vi "Fit Controls to Rect.vi"(4 "Error In":errorcluster, 6 "Rect":T1, 7 "GObjs":refnum<vi>[](array[refnum])) -> (0 "Error Out":errorcluster, 3 "GObjs":refnum<vi>[](array[refnum]))   [LabVIEW 2017]
doc: "Moves the front panel objects in GObjs so that their combined bounding rectangle is centred inside Rect."
uses:
  <vilib>/Utility/miscctls.llb/LVRectTypeDef.ctl
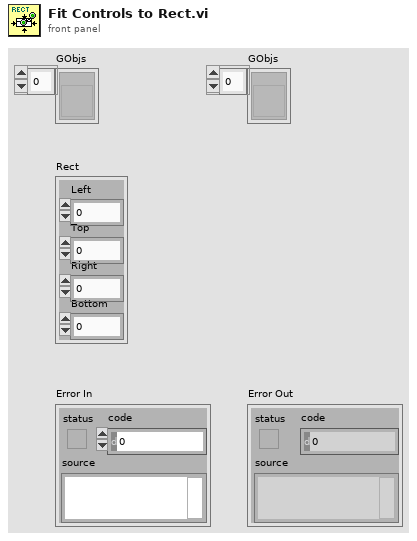
[diagram p1: front panel]
types:
  T1 = typedef "LVRectTypeDef.ctl" = cluster{"Left":i16, "Top":i16, "Right":i16, "Bottom":i16}
  T2 = cluster{"left":i16, "top":i16, "right":i16, "bottom":i16}
  T3 = typedef "LVPositionTypeDef.ctl" = cluster{"Left":i32, "Top":i32}
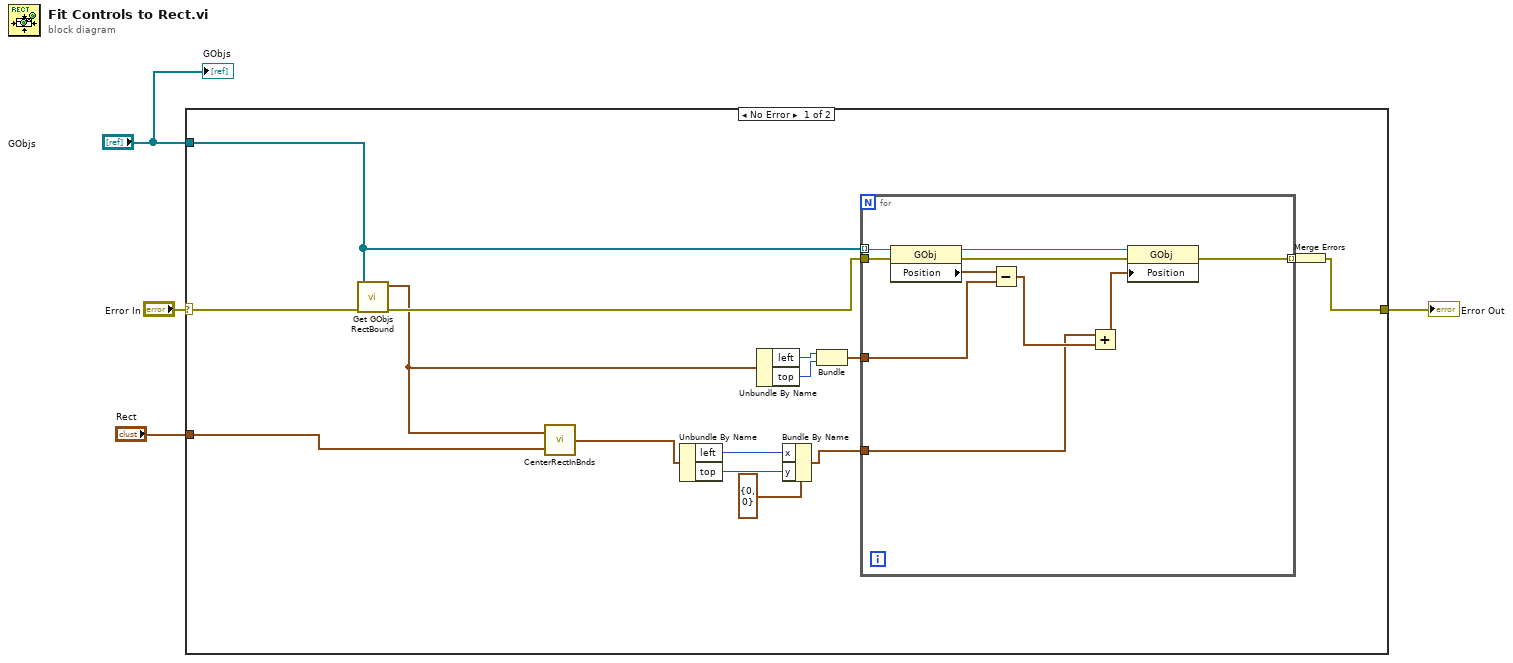
[diagram p0: block diagram]
diagram:
  n1 = case shown="No Error" "Error In" {
    selector: "Error In" -> [w19 w30]
    tunnel: [w11 w30] -> w4
    tunnel: "GObjs" -> [w18 _]
    tunnel: "Rect" -> [w10 _]
    frame No Error {
      n2 = call "Get GObjs RectBound.vi"("error in"=w19, "GObjs"=w18) -> ("error out"=w13:errorcluster, "Bound"=w9:T2)  [unwired: 8 in]
      n3 = call <vilib>:"CenterRectInBnds.vi"("bounds"=w10, "rect"=w9) -> ("centered rect"=w8:T2)
      n4 = Unbundle By Name(w8) -> ("left"=w6:i16, "top"=w7:i16)
      n5 = Unbundle By Name(w9) -> ("left"=w17:i16, "top"=w16:i16)
      n6 = Bundle By Name(cluster=cluster{"x":i32, "y":i32} {"x"=0, "y"=0} ("Point"), "x"=w6, "y"=w7) -> (w14:cluster{"x":i32, "y":i32})
      n7 = Bundle("left"=w17, "top"=w16) -> (w15:cluster{"left":i16, "top":i16})  [unwired: 1 in]
      n8 = for {
        tunnel: w18 -> [w29] mode=indexing
        tunnel: w15 -> [w22]
        tunnel: w14 -> [w20]
        tunnel: w13 -> [w25]
        tunnel: [w23] -> w12 mode=indexing
        n9 = property class="GObj"(reference=w29, error in=w25) -> (reference out=w28:refnum<vi>, error out=w24:errorcluster, "Position"=w27:T3)
        n10 = Subtract(x=w27, y=w22) -> (x-y=w26:T3)
        n11 = Add(x=w20, y=w26) -> (x+y=w21:T3)
        n12 = property class="GObj"(reference=w28, error in=w24, "Position"=w21) -> (error out=w23:errorcluster)  [unwired: 1 out]
      }
      n13 = Merge Errors(w12) -> (w11:errorcluster)
    }
    frame Error {
    }
  }
  "Error Out" <- w4
  "GObjs" <- "GObjs"
